vi "Logic_Config_Capture_Duration.vi"(4 "error in (no error)":errorcluster, 6 "Capture Duration (s)":dbl=5.0 format="%#_13g", 7 "Session Ref In":T1) -> (0 "error out":errorcluster, 3 "Session Ref Out":T1)   [LabVIEW 2023]
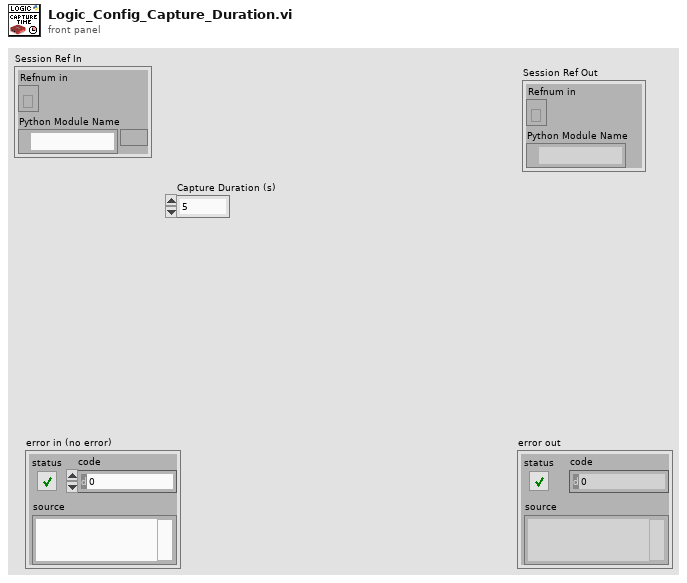
[diagram p1: front panel]
types:
  T1 = cluster{"Refnum in":refnum<k35>, "Python Module Name":path}
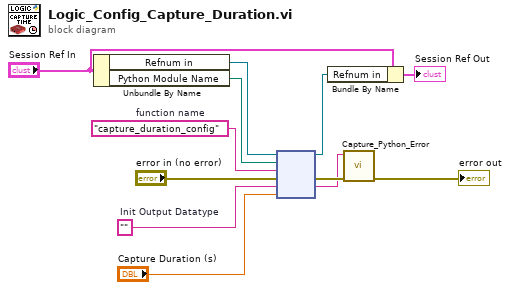
[diagram p0: block diagram]
diagram:
  w11 = "capture_duration_config"  # function name
  w10 = ""  # Init Output Datatype
  n1 = Unbundle By Name("Session Ref In") -> ("Refnum in"=w9:refnum<k35>, "Python Module Name"=w8:path)
  n2 = node(w9, w8, w11, "error in (no error)", w10, "Capture Duration (s)") -> (w6:refnum<k35>, w3:errorcluster, w1:string)  [unwired: 1 in, 2 out]
  n3 = Bundle By Name(cluster="Session Ref In", "Refnum in"=w6) -> (→"Session Ref Out":T1)
  n4 = call "Capture_Python_Error.vi"("error in (no error)"=w3, "Error Message (start with ERROR)"=w1) -> ("error out"=→"error out":errorcluster)  [unwired: 9 in]
